vi "数据写入database.vi"(9 "data":variant, 10 "columns":string[](array[string]), 11 "table":string) -> (1 "error out":errorcluster)   [LabVIEW 2016, in "斯坦道CODMn.lvlib"]
uses:
  <vilib>/Utility/sysdir.llb/System Directory Type.ctl
  <vilib>/Utility/error.llb/DialogType.ctl
  <vilib>/addons/database/Auxilliary.llb/DB Tools Transaction.ctl
  <vilib>/addons/database/Auxilliary.llb/DB Tools Isolation Level.ctl
  <vilib>/addons/database/Connection.llb/DB Tools Open Connec (String).vi
  <vilib>/addons/database/Connection.llb/Conn Execute.vi
  <vilib>/addons/database/Recordset.llb/Rec Destroy - Connection.vi
  <vilib>/addons/database/Recordset.llb/Rec Fetch Recordset Data (R).vi
  <vilib>/addons/database/Connection.llb/Conn Transaction.vi
  <vilib>/addons/database/NI_Database_API.lvlib
panel:
  out "为空？":bool
  in  "error in (no error)":errorcluster
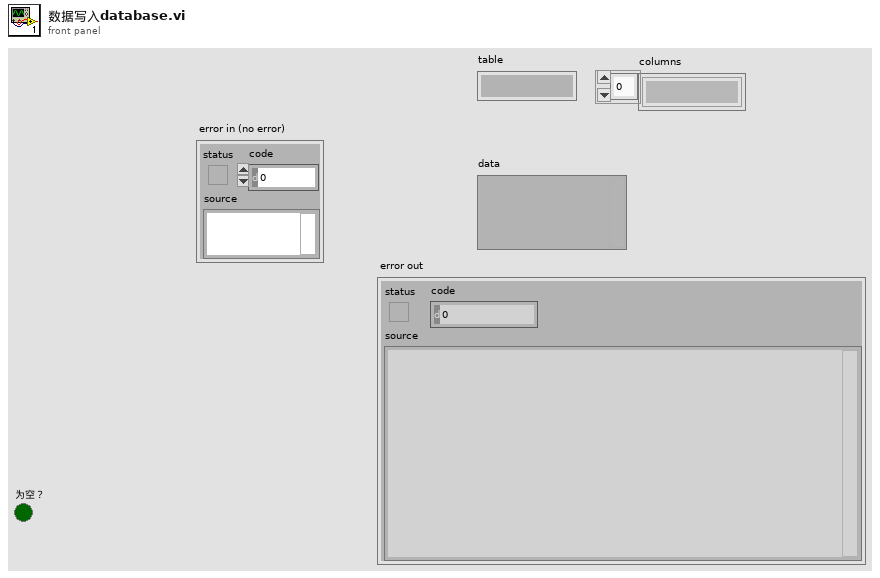
[diagram p1: front panel]
types:
  T1 = cluster{"时间":timestamp, "测量模式":string, "数据类型":string, "检测值":sgl, "单位":string, "数据标识":string, "因子编码":string, "标样参考值":sgl, "ORP-A":sgl, "ORP-B":sgl, "ORP-K":sgl, "COD滴定值":sgl, "高锰酸钾滴定数":sgl, "温度":sgl, "量程":sgl, "LastTime":timestamp, "序列号:":string}
  T2 = typedef "DialogType.ctl" = u16
  T3 = typedef "System Directory Type.ctl" = i32
  T4 = typedef "NI_Database_API.lvlib/Conn ObjectReference.ctl" = refnum<k1>
  T5 = typedef "NI_Database_API.lvlib/Rec ObjectReference.ctl" = refnum<k1>
  T6 = typedef "NI_Database_API.lvlib/DB Tools Transaction.ctl" = enum16{"begin", "commit", "rollback"}
  T7 = typedef "NI_Database_API.lvlib/DB Tools Isolation Level.ctl" = enum16{"chaos", "read uncommitted", "read committed", "repeatable read", "serializable"}
  T8 = cluster{"时间标识":timestamp, "设备":string, "日志信息":string}
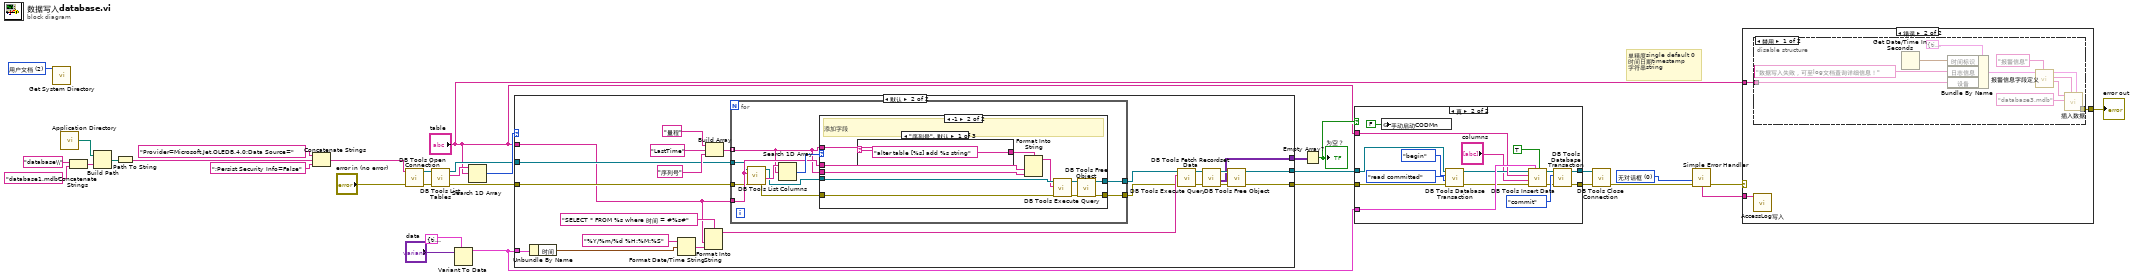
[diagram p0: block diagram]
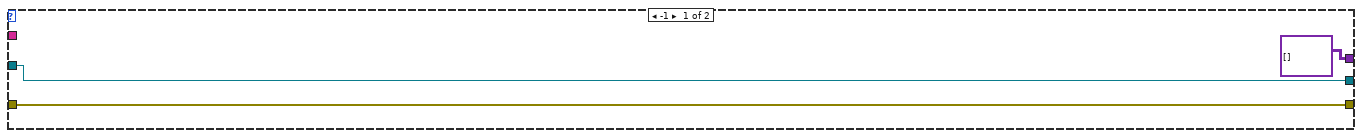
[diagram p4: hidden frame]
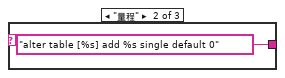
[diagram p6: hidden frame]
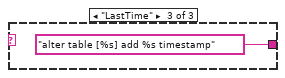
[diagram p7: hidden frame]
diagram:
  w9 = T2 0 items=["无对话框", "确定信息", "继续或停止信息", "确定信息＋警告", "继续/停止+警告"] ("type of dialog (OK msg:1)")
  w32 = T3 2 items=["用户目录"=0, "用户桌面"=1, "用户文档"=2, "用户应用程序数据"=3, "用户设置"=4, "用户临时目录"=5, "公共文档"=6, "公共应用程序数据"=7, "公共设置"=8, "公共缓存"=13, "系统核心库"=9, "系统安装库"=10, "应用程序文件"=11, "启动盘根目录"=12] ("system directory type")
  # "单精度single default 0\n时间日期timestamp\n字符串string"
  n1 = call <vilib>:"Get System Directory.vi"("system directory type"=w32) -> ()  [unwired: 10 in, 1 out]
  n2 = call <vilib>:"Application Directory.vi"() -> ("Application Directory"=w1:path)
  n3 = Concatenate Strings("database\\" ("condition"), "database1.mdb" ("字符串")) -> (w25:string)
  n4 = Build Path(base path=w1, name or relative path=w25) -> (appended path=w30:path)
  n5 = Path To String(path=w30) -> (string=w29:string)
  n6 = Concatenate Strings("Provider=Microsoft.Jet.OLEDB.4.0;Data Source=" ("condition"), w29, ";Persist Security Info=False" ("condition")) -> (w27:string)
  n7 = call-poly <vilib>:"DB Tools Open Connection.vi"("error in (no error)"="error in (no error)", "connection information"=w27) -> ("error out"=w23:errorcluster, "connection reference"=w24:T4)  [unwired: 6 in]
  n8 = call <vilib>:"DB Tools List Tables.vi"("error in (no error)"=w23, "connection reference"=w24) -> ("error out"=w17:errorcluster, "tables"=w22:string[], "connection reference out"=w18:T4)  [unwired: 3 in]
  n9 = Variant To Data(type=T1 {"时间"=timestamp(0 s since 1904-01-01), "测量模式"="", "数据类型"="", "检测值"=0.0, "单位"="", "数据标识"="", "因子编码"="", "标样参考值"=0.0, "ORP-A"=0.0, "ORP-B"=0.0, "ORP-K"=0.0, "COD滴定值"=0.0, "高锰酸钾滴定数"=0.0, "温度"=0.0, "量程"=0.0, "LastTime"=timestamp(0 s since 1904-01-01), "序列号:"=""} ("data"), Variant="data") -> (data=w10:T1)  [unwired: 1 in, 1 out]
  n10 = Search 1D Array(1D array=w22, element="table") -> (index of element=w19:i32)  [unwired: 1 in]
  n11 = case shown="默认" w19 {
    tunnel: [variant[][] [] ("recordset data") w46] -> w16
    tunnel: [w35 w53] -> w15
    tunnel: [w34 w52] -> w14
    tunnel: w18 -> [w35 w40]
    tunnel: w17 -> [w34 w39]
    tunnel: "table" -> [_ w38]
    tunnel: w10 -> [_ w47]
    frame -1 {
    }
    frame Default {
      n12 = Unbundle By Name(w47) -> ("时间"=w50:timestamp)
      n13 = Format Date/Time String(time format string (%c)="%Y/%m/%d %H:%M:%S" ("时间格式字符串(%c)"), seconds (now)=w50) -> (date/time string=w48:string)  [unwired: 1 in]
      n14 = Format Into String(format string="SELECT * FROM %s where 时间 = #%s#" ("格式字符串"), w38, w48) -> (resulting string=w51:string)  [unwired: 2 in, 1 out]
      n15 = Build Array("量程" ("元素"), "LastTime" ("元素"), "序列号" ("元素")) -> (w44:string[])
      n16 = for {
        tunnel: w38 -> [w65]
        tunnel: w44 -> [w62] mode=indexing
        tunnel: [w61] -> w37
        tunnel: [w60] -> w36
        tunnel: w40 -> [w59]
        tunnel: w39 -> [w58]
        n17 = call <vilib>:"DB Tools List Columns.vi"("error in (no error)"=w58, "table"=w65, "connection reference"=w59) -> ("error out"=w63:errorcluster, "columns"=w67:string[], "connection reference out"=w64:T4)  [unwired: 1 in, 1 out]
        n18 = Search 1D Array(1D array=w67, element=w62) -> (index of element=w66:i32)  [unwired: 1 in]
        n19 = case shown="-1" w66 {
          tunnel: w64 -> [w69 w78]
          tunnel: w63 -> [w68 w77]
          tunnel: w62 -> [_ w76]
          tunnel: [w69 w74] -> w61
          tunnel: [w68 w73] -> w60
          tunnel: w65 -> [_ w72]
          tunnel: w62 -> [_ w71]
          frame 0, Default {
          }
          frame -1 {
            # "添加字段"
            n20 = case shown="\"序列号\", 默认" w71 {
              tunnel: ["alter table [%s] add %s string" "alter table [%s] add %s single default 0" "alter table [%s] add %s timestamp"] -> w70
              frame "序列号", Default {
              }
              frame "量程" {
              }
              frame "LastTime" {
              }
            }
            n21 = Format Into String(format string=w70, w72, w76) -> (resulting string=w75:string)  [unwired: 2 in, 1 out]
            n22 = call-poly <vilib>:"DB Tools Execute Query.vi"("error in (no error)"=w77, "SQL query"=w75, "connection reference"=w78) -> ("error out"=w79:errorcluster, "recordset reference"=w80:T5)  [unwired: 5 in]
            n23 = call-poly <vilib>:"DB Tools Free Object.vi"("error in (no error)"=w79, "recordset reference"=w80) -> ("error out"=w73:errorcluster, "connection reference"=w74:T4)  [unwired: 8 in]
          }
        }
      }
      n24 = call-poly <vilib>:"DB Tools Execute Query.vi"("error in (no error)"=w36, "SQL query"=w51, "connection reference"=w37) -> ("error out"=w54:errorcluster, "recordset reference"=w57:T5)  [unwired: 5 in]
      n25 = call-poly <vilib>:"DB Tools Fetch Recordset Data.vi"("error in (no error)"=w54, "recordset reference"=w57) -> ("error out"=w55:errorcluster, "recordset data"=w46:variant[][], "recordset reference out"=w56:T5)  [unwired: 3 in]
      n26 = call-poly <vilib>:"DB Tools Free Object.vi"("error in (no error)"=w55, "recordset reference"=w56) -> ("error out"=w52:errorcluster, "connection reference"=w53:T4)  [unwired: 8 in]
    }
  }
  n27 = Empty Array?(array=w16) -> (empty?=w11:bool)
  "为空？" <- w11
  n28 = case shown="真" w11 {
    tunnel: "table" -> [_ w99]
    tunnel: w10 -> [_ w100]
    tunnel: w14 -> [w84 w93]
    tunnel: w15 -> [w85 w94]
    tunnel: [w85 w88] -> w21
    tunnel: [w84 w87] -> w20
    frame False {
    }
    frame True {
      n29 = global write "CODMN外部API.vi" "手动启动CODMn"(FALSE ("手动启动CODMn")) -> ()
      n30 = call-poly <vilib>:"DB Tools Database Transaction.vi"("error in (no error)"=w93, "isolation level (chaos)"=DB_Tools_Isolation_Level."read committed", "operation (begin)"=DB_Tools_Transaction."begin", "connection reference"=w94) -> ("error out"=w91:errorcluster, "connection reference out"=w92:T4)  [unwired: 2 in]
      n31 = call <vilib>:"DB Tools Insert Data.vi"("create table? (F)"=TRUE, "data"=w100, "error in (no error)"=w91, "columns"="columns", "table"=w99, "connection reference"=w92) -> ("error out"=w89:errorcluster, "connection reference out"=w90:T4)  [unwired: 4 in]
      n32 = call-poly <vilib>:"DB Tools Database Transaction.vi"("error in (no error)"=w89, "operation (begin)"=DB_Tools_Transaction."commit", "connection reference"=w90) -> ("error out"=w87:errorcluster, "connection reference out"=w88:T4)  [unwired: 3 in]
    }
  }
  n33 = call <vilib>:"DB Tools Close Connection.vi"("error in (no error)"=w20, "connection reference"=w21) -> ("error out"=w7:errorcluster)  [unwired: 5 in]
  n34 = call <vilib>:"Simple Error Handler.vi"("type of dialog (OK msg:1)"=w9, "error in (no error)"=w7) -> ("error out"=w8:errorcluster, "message"=w4:string)  [unwired: 3 in, 3 out]
  n35 = case shown="错误" w8 {
    tunnel: "table" -> [_ w104]
    tunnel: [_ w103] -> w5
    tunnel: w4 -> [_ w102]
    frame No Error {
    }
    frame Error {
      n36 = call "AccessLog写入.vi"("Log"=w102) -> ()  [unwired: 11 in]
      n37 = disable-structure shown="禁用" {
        disable-tunnel: w104 -> [w113 _]
        disable-tunnel: [w106 _] -> w103
        frame Disabled {
          n38 = Get Date/Time In Seconds() -> (seconds since 1Jan1904=w114:timestamp)
          n39 = Bundle By Name(cluster=T8 {"时间标识"=timestamp(0 s since 1904-01-01), "设备"="氨氮", "日志信息"=""} ("data in"), "时间标识"=w114, "日志信息"="数据写入失败，可至log文档查询详细信息！" ("table输入"), "设备"=w113) -> (w107:T8)
          n40 = call "报警信息字段定义.vi"("table输入"="报警信息", "data in"=w107) -> ("table输出"=w110:string, "columns"=w111:string[], "data out"=w112:T8)  [unwired: 7 in]
          n41 = call "插入数据.vi"("data"=w112, "columns"=w111, "database"="database3.mdb", "table"=w110) -> ("error out"=w106:errorcluster)  [unwired: 7 in]
        }
        frame Enabled {
        }
      }
    }
  }
  "error out" <- w5
